vi "AquireBgImages.vi"(0 "object in":refnum<class "Application.lvclass">, 2 "Number of Background Images":i32, 3 "BG Images Folder Name":path, 5 "error in (no error)":errorcluster) -> (14 "object out":refnum<class "Application.lvclass">, 19 "error out":errorcluster)   [LabVIEW 2021, in "Application.lvclass"]
uses:
  Application.lvclass
  Application.lvclass/Application.ctl
  Hamamatsu_class/Hamamatsu.lvclass
  AD2_SDK_class/AD2_SDK.lvclass
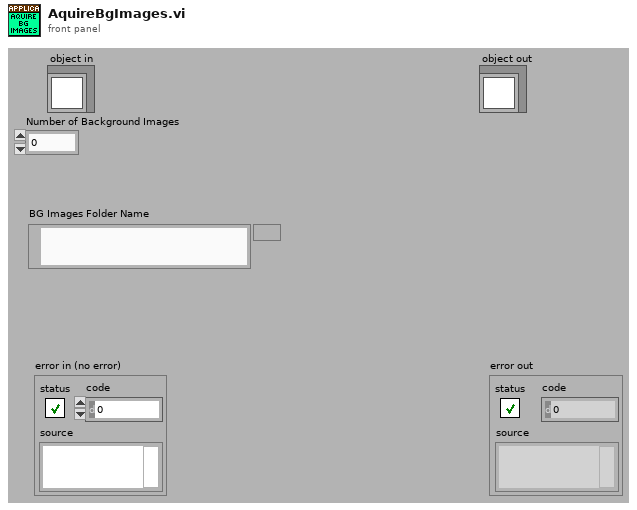
[diagram p1: front panel]
types:
  T1 = typedef "IMAQ Image.ctl" = refnum<image>
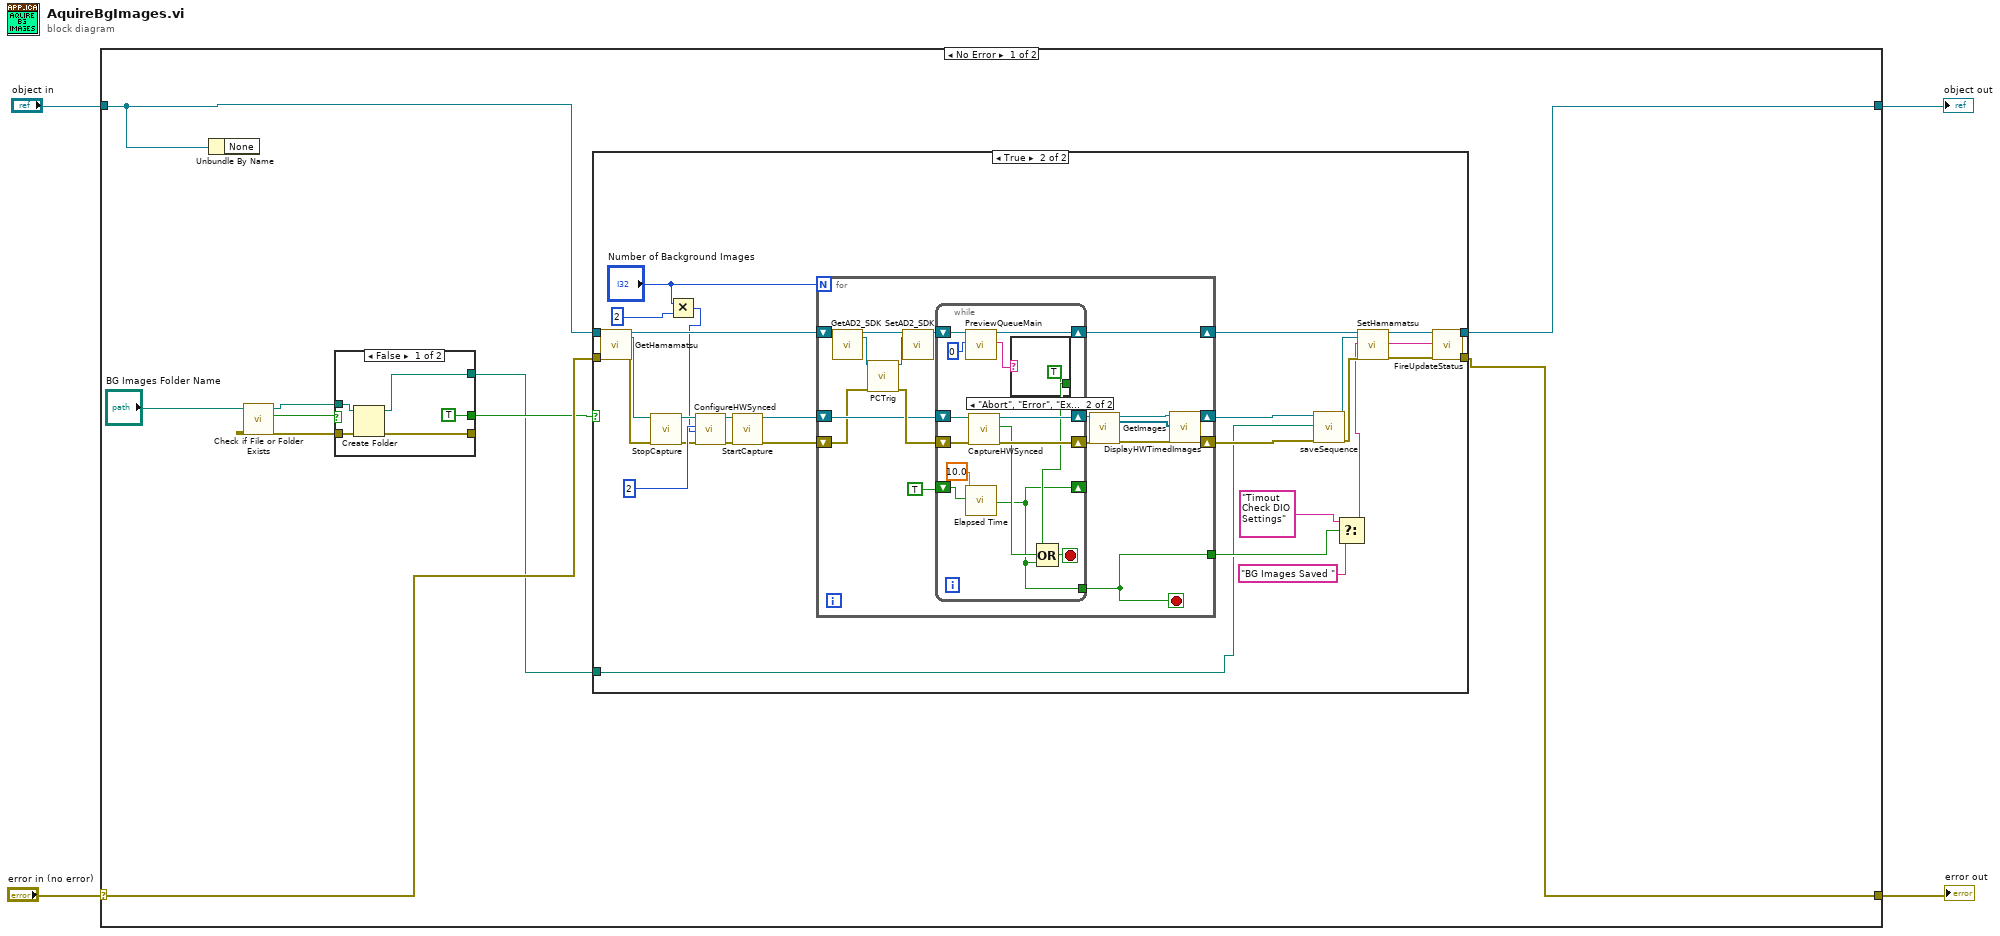
[diagram p0: block diagram]
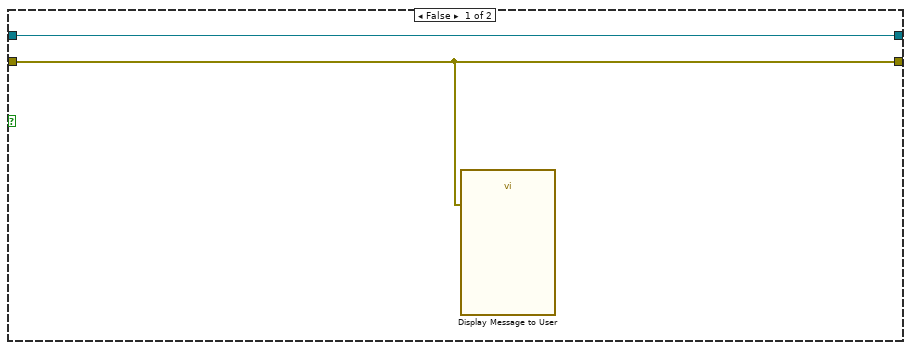
[diagram p2: hidden frame]
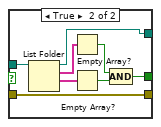
[diagram p4: hidden frame]
diagram:
  n1 = case shown="No Error" "error in (no error)" {
    selector: "error in (no error)" -> [w10 w93]
    tunnel: [w9 w93] -> w3
    tunnel: [w8 w92] -> w1
    tunnel: "object in" -> [w7 w92]
    frame No Error {
      n2 = Unbundle By Name(w7) -> ()  [unwired: 1 out]
      n3 = call <vilib>:"Check if File or Folder Exists.vi"("path"="BG Images Folder Name") -> ("error out"=w14:errorcluster, "file or folder exists?"=w12:bool, "dup path"=w13:path)  [unwired: 8 in]
      n4 = case shown="False" w12 {
        tunnel: w13 -> [w83 w87]
        tunnel: [w82 w85] -> w5
        tunnel: w14 -> [w81 w84]
        tunnel: [w80 w84] -> _
        tunnel: [TRUE w86] -> w6
        frame False {
          n5 = Create Folder(path (use dialog)=w83, error in=w81) -> (created path=w82:path, error out=w80:errorcluster)  [unwired: 1 in, 1 out]
        }
        frame True {
          n6 = List Folder(path=w87) -> (path out=w85:path, filenames=w89:string[], folder names=w88:string[])  [unwired: 3 in, 1 out]
          n7 = Empty Array?(array=w89) -> (empty?=w91:bool)
          n8 = Empty Array?(array=w88) -> (empty?=w90:bool)
          n9 = Compound Arithmetic op=AND(w91, w90) -> (w86:bool)
        }
      }
      n10 = case shown="True" w6 {
        tunnel: w10 -> [w15 w21]
        tunnel: [w15 w20] -> w9
        tunnel: [w16 w19] -> w8
        tunnel: w7 -> [w16 w18]
        tunnel: w5 -> [_ w17]
        frame False {
          n11 = call "Display Message to User"("error in (no error)"=w15) -> ()  [unwired: 9 in, 2 out]
        }
        frame True {
          n12 = call-dynamic "GetHamamatsu.vi"("object in"=w18, "error in (no error)"=w21) -> ("object out"=w38:refnum<class "Application.lvclass">, "Hamamatsu"=w37:refnum<class "Hamamatsu.lvclass">, "error out"=w24:errorcluster)  [unwired: 15 in]
          n13 = call-dynamic "StopCapture.vi"("object in"=w37, "error in (no error)"=w24) -> ("object out"=w45:refnum<class "Hamamatsu.lvclass">, "error out"=w41:errorcluster)  [unwired: 16 in]
          n14 = Multiply(x="Number of Background Images", y=2) -> (x*y=w35:i32)
          n15 = call-dynamic "ConfigureHWSynced.vi"("object in"=w45, "FramesPerAquisionCycle"=2, "CameraBufferSize"=w35, "error in (no error)"=w41) -> ("object out"=w43:refnum<class "Hamamatsu.lvclass">, "error out"=w44:errorcluster)  [unwired: 14 in]
          n16 = call-dynamic "StartCapture.vi"("object in"=w43, "error in (no error)"=w44) -> ("object out"=w40:refnum<class "Hamamatsu.lvclass">, "error out"=w39:errorcluster)  [unwired: 16 in]
          n17 = for {
            N: "Number of Background Images" -> [_]
            shift-right: [w47] -> w32
            shift-left: w38 -> [w50]
            shift-right: [w49] -> w31
            shift-left: w40 -> [w52]
            tunnel: [w46] -> w22
            shift-right: [w48] -> w28
            shift-left: w39 -> [w51]
            stop <- w46 stop-if-true
            n18 = call-dynamic "GetAD2_SDK.vi"("object in"=w50) -> ("object out"=w60:refnum<class "Application.lvclass">, "AD2_SDK"=w61:refnum<class "AD2_SDK.lvclass">)  [unwired: 16 in, 1 out]
            n19 = call-dynamic "PCTrig.vi"("object in"=w61, "error in (no error)"=w51) -> ("object out"=w62:refnum<class "AD2_SDK.lvclass">, "error out"=w53:errorcluster)  [unwired: 16 in]
            n20 = call-dynamic "SetAD2_SDK.vi"("object in"=w60, "AD2_SDK"=w62) -> ("object out"=w54:refnum<class "Application.lvclass">)  [unwired: 16 in, 1 out]
            n21 = while {
              shift-right: [w75] -> w63
              shift-left: w52 -> [w77]
              shift-right: [w74] -> w59
              shift-left: w53 -> [w76]
              tunnel: [w67] -> w46
              shift-right: [w67] -> _
              shift-left: TRUE ("Time has Elapsed") -> [w66]
              shift-right: [w72] -> w47
              shift-left: w54 -> [w73]
              stop <- w68 stop-if-true
              n22 = call-dynamic "PreviewQueueMain.vi"("object in"=w73, "timeout in ms (-1)"=0) -> ("object out"=w72:refnum<class "Application.lvclass">, "Message"=w71:string)  [unwired: 14 in, 2 out]
              n23 = call "Elapsed Time"("Time Target (s)"=10.0, "Reset"=w66) -> ("Time has Elapsed"=w67:bool)  [unwired: 10 in, 7 out]
              n24 = call-dynamic "CaptureHWSynced.vi"("object in"=w77, "error in (no error)"=w76) -> ("object out"=w75:refnum<class "Hamamatsu.lvclass">, "AllFramesAvailable?"=w69:bool, "error out"=w74:errorcluster)  [unwired: 13 in, 2 out]
              n25 = case shown="\"Abort\", \"Error\", \"Exit\"" w71 {
                tunnel: [_ TRUE] -> w70
                frame "False", Default {
                }
                frame "Abort", "Error", "Exit" {
                }
              }
              n26 = Compound Arithmetic op=OR(w70, w69, w67) -> (w68:bool)
            }
            n27 = call-dynamic "GetImages.vi"("object in"=w63, "error in (no error)"=w59) -> ("object out"=w57:refnum<class "Hamamatsu.lvclass">, "HWSyncedImages"=w55:T1[], "error out"=w56:errorcluster)  [unwired: 15 in]
            n28 = call-dynamic "DisplayHWTimedImages.vi"("object in"=w57, "HWSyncedImages"=w55, "error in (no error)"=w56) -> ("object out"=w49:refnum<class "Hamamatsu.lvclass">, "error out"=w48:errorcluster)  [unwired: 15 in]
          }
          n29 = call-dynamic "saveSequence.vi"("object in"=w31, "folder path"=w17, "error in (no error)"=w28) -> ("object out"=w30:refnum<class "Hamamatsu.lvclass">, "error out"=w29:errorcluster)  [unwired: 13 in, 2 out]
          n30 = Select(t="Timout Check DIO Settings", s=w22, f="BG Images Saved " ("Status")) -> (s? t:f=w25:string)
          n31 = call-dynamic "SetHamamatsu.vi"("object in"=w32, "Hamamatsu"=w30, "error in (no error)"=w29) -> ("object out"=w33:refnum<class "Application.lvclass">, "error out"=w23:errorcluster)  [unwired: 15 in]
          n32 = call-dynamic "FireUpdateStatus.vi"("object in"=w33, "Status"=w25, "error in (no error)"=w23) -> ("object out"=w19:refnum<class "Application.lvclass">, "error out"=w20:errorcluster)  [unwired: 15 in]
        }
      }
    }
    frame Error {
    }
  }
  "error out" <- w3
  "object out" <- w1
